vi "create files.vi"(8 "error in":errorcluster, 10 "create files":bool, 11 "base path":path) -> (0 "error out":errorcluster, 3 "refnums":T1)   [LabVIEW 2017]
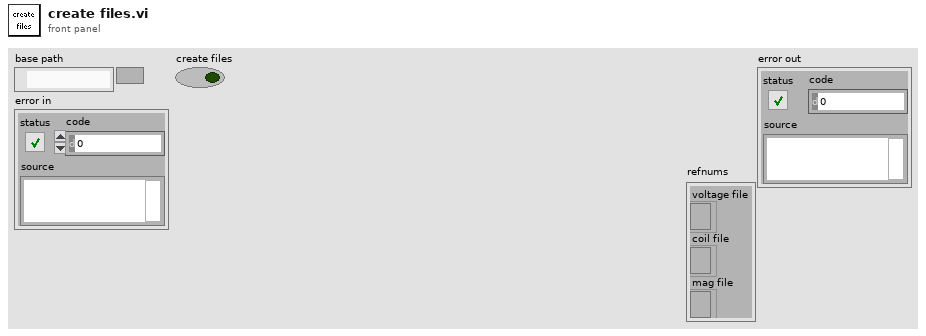
[diagram p1: front panel]
types:
  T1 = cluster{"voltage file":refnum<file>, "coil file":refnum<file>, "mag file":refnum<file>}
  T2 = enum16{"open", "replace", "create", "open or create", "replace or create", "replace or create with confirmation"}
  T3 = cluster{"refnum out":refnum<file>, "refnum out":refnum<file>, "refnum out":refnum<file>}
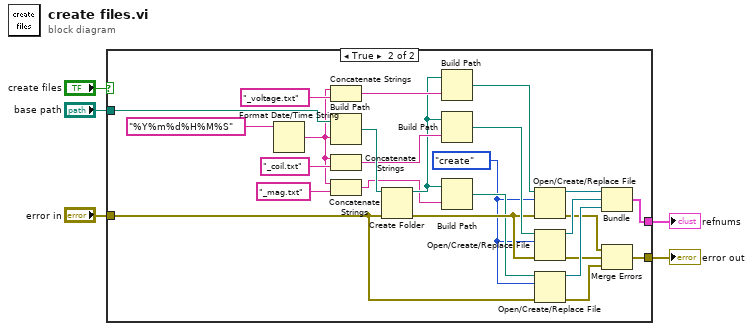
[diagram p0: block diagram]
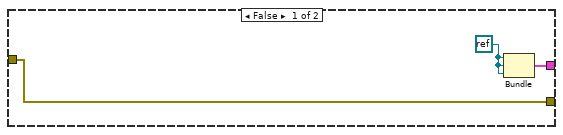
[diagram p2: hidden frame]
diagram:
  n1 = case shown="True" "create files" {
    tunnel: "base path" -> [_ w33]
    tunnel: "error in" -> [w8 w22]
    tunnel: [w6 w14] -> w3
    tunnel: [w8 w10] -> w2
    frame False {
      w7 = refnum<k0> refnum
      n2 = Bundle(w7, w7, w7) -> (w6:cluster{refnum<k0>, refnum<k0>, refnum<k0>})  [unwired: 1 in]
    }
    frame True {
      w9 = T2."create" ("operation (0:open)")
      n3 = Format Date/Time String(time format string (%c)="%Y%m%d%H%M%S") -> (date/time string=w19:string)  [unwired: 2 in]
      n4 = Concatenate Strings(w19, "_voltage.txt" ("string")) -> (w29:string)
      n5 = Build Path(base path=w33, name or relative path=w19) -> (appended path=w31:path)
      n6 = Concatenate Strings(w19, "_coil.txt" ("string")) -> (w26:string)
      n7 = Concatenate Strings(w19, "_mag.txt" ("string")) -> (w18:string)
      n8 = Create Folder(path (use dialog)=w31, error in=w22) -> (created path=w21:path, error out=w24:errorcluster)  [unwired: 1 in, 1 out]
      n9 = Build Path(base path=w21, name or relative path=w29) -> (appended path=w28:path)
      n10 = Build Path(base path=w21, name or relative path=w26) -> (appended path=w25:path)
      n11 = Build Path(base path=w21, name or relative path=w18) -> (appended path=w23:path)
      n12 = Open/Create/Replace File(file path (use dialog)=w28, error in=w24, operation (0:open)=w9) -> (refnum out=w17:refnum<file>, error out=w13:errorcluster)  [unwired: 3 in, 1 out]
      n13 = Open/Create/Replace File(file path (use dialog)=w25, error in=w24, operation (0:open)=w9) -> (refnum out=w16:refnum<file>, error out=w12:errorcluster)  [unwired: 3 in, 1 out]
      n14 = Open/Create/Replace File(file path (use dialog)=w23, error in=w22, operation (0:open)=w9) -> (refnum out=w15:refnum<file>, error out=w11:errorcluster)  [unwired: 3 in, 1 out]
      n15 = Bundle("refnum out"=w17, "refnum out"=w16, "refnum out"=w15) -> (w14:T3)  [unwired: 1 in]
      n16 = Merge Errors(w13, w12, w11) -> (w10:errorcluster)
    }
  }
  "refnums" <- w3
  "error out" <- w2
